vi "IsFactor.vi"(9 "Numeric Control 2":dbl, 10 "Numeric Control":dbl) -> (2 "Boolean":bool)   [LabVIEW 2012]
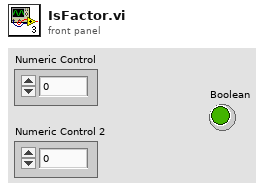
[diagram p1: front panel]
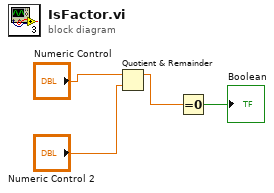
[diagram p0: block diagram]
diagram:
  n1 = Quotient & Remainder(x="Numeric Control", y="Numeric Control 2") -> (x-y*floor(x/y)=w4:dbl)  [unwired: 1 out]
  n2 = Equal To 0?(x=w4) -> (x = 0?=→"Boolean":bool)
